vi "FT_Set_Baud_Rate.vi"(1 "Baud Rate":u32, 2 "Handle":u32) -> (0 "FT_Status":u32)   [LabVIEW 2014]
uses:
  FTD2XX.DLL
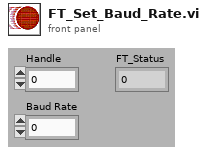
[diagram p1: front panel]
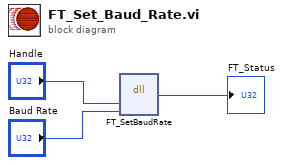
[diagram p0: block diagram]
diagram:
  n1 = dll-call lib="FTD2XX.dll" fn="FT_SetBaudRate"("Handle"="Handle", "BaudRate"="Baud Rate") -> ("FT_Status"=→"FT_Status":u32)  [unwired: 5 in, 2 out]
